vi "Basic MQTT Subscribe.vi"() -> ()   [LabVIEW 2017]
uses:
  <vilib>/LabVIEW Open Source Project/MQTT Broker/Client/Client.lvclass/Client.ctl
  <vilib>/LabVIEW Open Source Project/MQTT Broker/Control Packets/ControlPacket/ControlPacket.lvclass/ControlPacket.ctl
  <vilib>/LabVIEW Open Source Project/MQTT Broker/Client/Client.lvclass
  C:/Program Files (x86)/National Instruments/LabVIEW 2017/vi.lib/LabVIEW Open Source Project/MQTT Broker/MQTT_Base/MQTT_Base.lvclass
  <vilib>/LabVIEW Open Source Project/MQTT Broker/Control Packets/PUBLISH/PUBLISH.lvclass
  C:/Program Files (x86)/National Instruments/LabVIEW 2017/vi.lib/LabVIEW Open Source Project/MQTT Broker/Control Packets/ControlPacket/ControlPacket.lvclass
  <vilib>/LabVIEW Open Source Project/MQTT Broker/MQTT_Base/MQTT_Base.lvclass
  <vilib>/LabVIEW Open Source Project/MQTT Broker/Control Packets/ControlPacket/ControlPacket.lvclass
panel:
  out "Payload":u8[](array[numeric]) format="%08b"
  out "error out":errorcluster
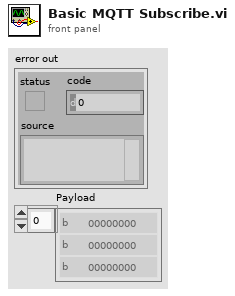
[diagram p1: front panel]
types:
  T1 = typedef "MQTT Server.lvlib/Client.lvclass/Public Events -- cluster.ctl" = cluster{"Connection Status":refnum<user-event>, "Connected":refnum<user-event>, "Application Message":refnum<user-event>}
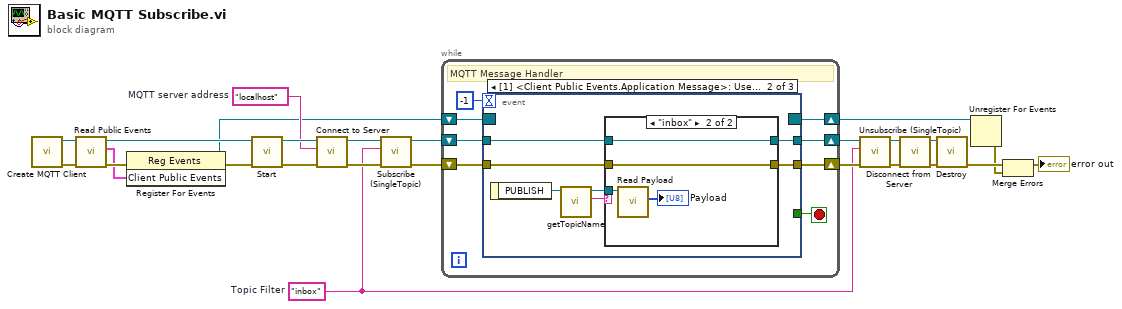
[diagram p0: block diagram]
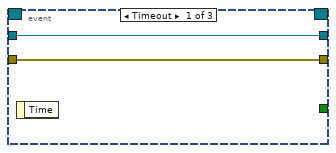
[diagram p2: hidden frame]
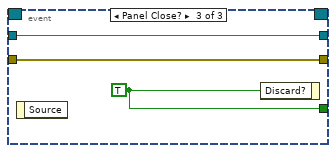
[diagram p4: hidden frame]
diagram:
  w1 = "inbox"  # Topic Filter
  w17 = "localhost"  # MQTT server address
  n1 = call <vilib>:"Create MQTT Client.vi"() -> ("error out"=w21:errorcluster, "Client out"=w23:refnum<class "Client.lvclass">)  [unwired: 10 in]
  n2 = call <vilib>:"Read Public Events.vi"("error in (no error)"=w21, "Client in"=w23) -> ("error out"=w20:errorcluster, "Client Public Events"=w18:T1, "Client out"=w22:refnum<class "Client.lvclass">)  [unwired: 7 in]
  n3 = register-events(error in=w20, w18) -> (reference out=w14:refnum<event-registration>, error out=w19:errorcluster)  [unwired: 1 in]
  n4 = call <vilib>:"Start.vi"("error in (no error)"=w19, "MQTT_Base in"=w22) -> ("error out"=w24:errorcluster, "MQTT_Base out"=w25:refnum<class "Client.lvclass">)  [unwired: 7 in, 1 out]
  n5 = call <vilib>:"Connect to Server.vi"("error in (no error)"=w24, "address (localhost)"=w17, "Client in"=w25) -> ("error out"=w7:errorcluster, "Client out"=w9:refnum<class "Client.lvclass">)  [unwired: 5 in, 2 out]
  n6 = call <vilib>:"Subscribe (SingleTopic).vi"("error in (no error)"=w7, "Topic Filter"=w1, "MQTT_Base in"=w9) -> ("error out"=w6:errorcluster, "MQTT_Base out"=w8:refnum<class "Client.lvclass">)  [unwired: 7 in]
  n7 = while {
    shift-right: [w30] -> w5
    shift-left: w8 -> [w32]
    shift-right: [w29] -> w3
    shift-left: w6 -> [w31]
    shift-right: [w26] -> w13
    shift-left: w14 -> [w27]
    stop <- w28 stop-if-true
    # "MQTT Message Handler"
    n8 = event shown="[1] <Client Public Events.Application Message>: User Event" {
      selector: w27 -> [_ _ _]
      dyn-events: [_ _ _] -> w26
      timeout: -1 -> [_ _ _]
      tunnel: w32 -> [w35 w40 w51]
      tunnel: w31 -> [w34 w37 w50]
      tunnel: [w35 w39 w51] -> w30
      tunnel: [w34 w38 w50] -> w29
      tunnel: [_ _ w49] -> w28
      event Timeout {
        n9 = event-data() -> ()  [unwired: 1 in, 1 out]
      }
      event User Event {
        n10 = event-data() -> ("PUBLISH"=w42:refnum<class "PUBLISH.lvclass">)  [unwired: 1 in]
        n11 = call <vilib>:"getTopicName.vi"("PUBLISH in"=w42) -> ("Topic"=w36:string, "PUBLISH out"=w41:refnum<class "PUBLISH.lvclass">)  [unwired: 8 in, 1 out]
        n12 = case shown="\"inbox\"" w36 {
          tunnel: w41 -> [_ w48]
          tunnel: w40 -> [w44 w47]
          tunnel: [w44 w47] -> w39
          tunnel: [w43 w46] -> w38
          tunnel: w37 -> [w43 w46]
          frame Default {
          }
          frame "inbox" {
            n13 = call <vilib>:"Read Payload.vi"("ControlPacket in"=w48) -> ("Payload"=→"Payload":u8[])  [unwired: 9 in, 1 out]
          }
        }
      }
      event Panel Close? {
        w49 = TRUE ("Discard?")
        n14 = event-data() -> ()  [unwired: 1 in, 1 out]
        n15 = event-data("Discard?"=w49) -> ()  [unwired: 1 in, 1 out]
      }
    }
  }
  n16 = call <vilib>:"Unsubscribe (SingleTopic).vi"("error in (no error)"=w3, "Topic Filter"=w1, "MQTT_Base in"=w5) -> ("error out"=w2:errorcluster, "MQTT_Base out"=w4:refnum<class "Client.lvclass">)  [unwired: 7 in]
  n17 = call <vilib>:"Disconnect from Server.vi"("error in (no error)"=w2, "Client in"=w4) -> ("error out"=w16:errorcluster, "Client out"=w15:refnum<class "Client.lvclass">)  [unwired: 7 in, 1 out]
  n18 = call-dynamic "Destroy.vi"("error in (no error)"=w16, "MQTT_Base in"=w15) -> ("error out"=w12:errorcluster)  [unwired: 8 in, 1 out]
  n19 = Unregister For Events(event registration refnum=w13) -> (error out=w10:errorcluster)  [unwired: 1 in]
  n20 = Merge Errors(w12, w10) -> (→"error out":errorcluster)
